vi "PXI_Host_I32_Read_NewMethod_Benchmark.vi"() -> ()   [LabVIEW 2018]
uses:
  <vilib>/Platform/TimedLoop/XDataNode/timing_clust.ctl
  <vilib>/Platform/TimedLoop/XDataNode/nitl_modes.ctl
  <vilib>/Platform/TimedLoop/XDataNode/wakeup.ctl
  cRIO RT/FPGA Bitfile Register Operations/Scalar IO Operations/Utilities/Find Register Offset.vi
  cRIO RT/FPGA Bitfile Register Operations/Scalar IO Operations/SubVIs/Check Register Data Store.vi
  cRIO RT/FPGA Bitfile Register Operations/Scalar IO Operations/Error Handling/Error 6001.vi
  cRIO RT/FPGA Bitfile Register Operations/Scalar IO Operations/Error Handling/Error 6000.vi
  cRIO RT/FPGA Bitfile Register Operations/Scalar IO Operations/Error Handling/Error 6002.vi
  cRIO RT/FPGA Bitfile Register Operations/Scalar IO Operations/Error Handling/Error 6003.vi
  <vilib>/FPGAPlugInAG/Dynamic/niLvFpga_Close_Dynamic.vi
  <vilib>/platform/TimedLoop/XDataNode/XDataNode.xnode
  <vilib>/rvi/interface/nirviCloseFPGA/nirviCloseFPGA.xnode
  cRIO RT/FPGA Bitfile Register Operations/Scalar IO Operations/Read Methods/Read Data Register/Instances/Read I32.vi
  cRIO RT/FPGA Bitfile Register Operations/Scalar IO Operations/FPGA Register IO.lvlib
  <vilib>/Platform/TimedLoop/XDataNode/XDNodeRunTimeDep.lvlib
panel:
  out "Waveform Graph":dbl[](graph)
  out "Standard Dev":dbl
  out "Arithmetic Mean":dbl
  out "Maximum":dbl
  out "Value out":i32
  out "error out":errorcluster
  # "Recorded time"
  # "3.37551E-5"
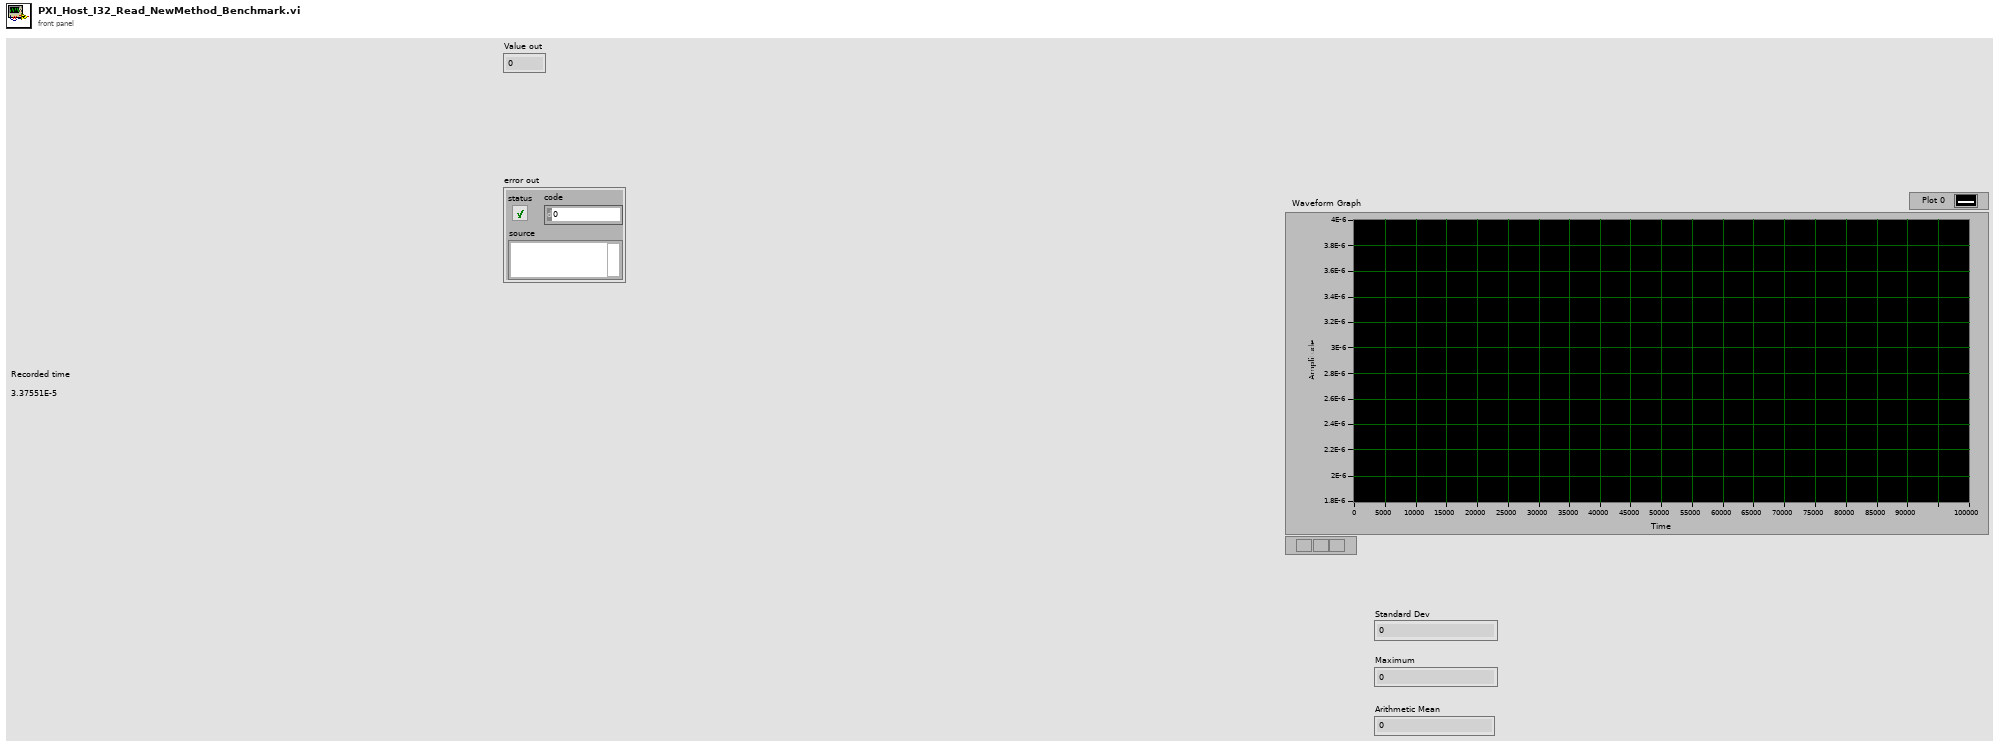
[diagram p1: front panel]
types:
  T1 = typedef "XDNodeRunTimeDep.lvlib/timing_clust.ctl" = cluster{"Expected End [f-1]":u64, "Actual End [f-1]":u64, "Finished Late? [f-1]":bool, "Expected End [i-1]":u64, "Actual End [i-1]":u64, "Finished Late? [i-1]":bool, "Expected Start [i]":u64, "Actual Start [i]":u64, "Expected Start [f]":u64, "Actual Start [f]":u64, "Source Name":string, "Structure Name":string, "Period":i64, "Deadline":i64, "Offset":i64, "Start":i64, "Priority":i32, "Timeout":i32, "Mode":T2, "Wakeup Reason":T3, "Error":errorcluster, "Source Type":string, "Secondary Source Type":string, "Global End Time":u64, "Global Start Time":u64, "Frame Duration":u64, "Iteration Duration":u64, "Assigned CPU":i32, "I/O Scan Engine Mode":u32}
  T2 = typedef "XDNodeRunTimeDep.lvlib/nitl_modes.ctl" = enum32{"No Change", "Process missed periods, maintain original phase", "Discard missed periods, maintain original phase", "Process missed periods, ignore original phase", "Discard missed periods, ignore original phase"}
  T3 = typedef "XDNodeRunTimeDep.lvlib/wakeup.ctl" = enum32{"Normal", "Aborted", "Asynchronous wakeup", "Timing source error", "Timed loop error", "Timeout"}
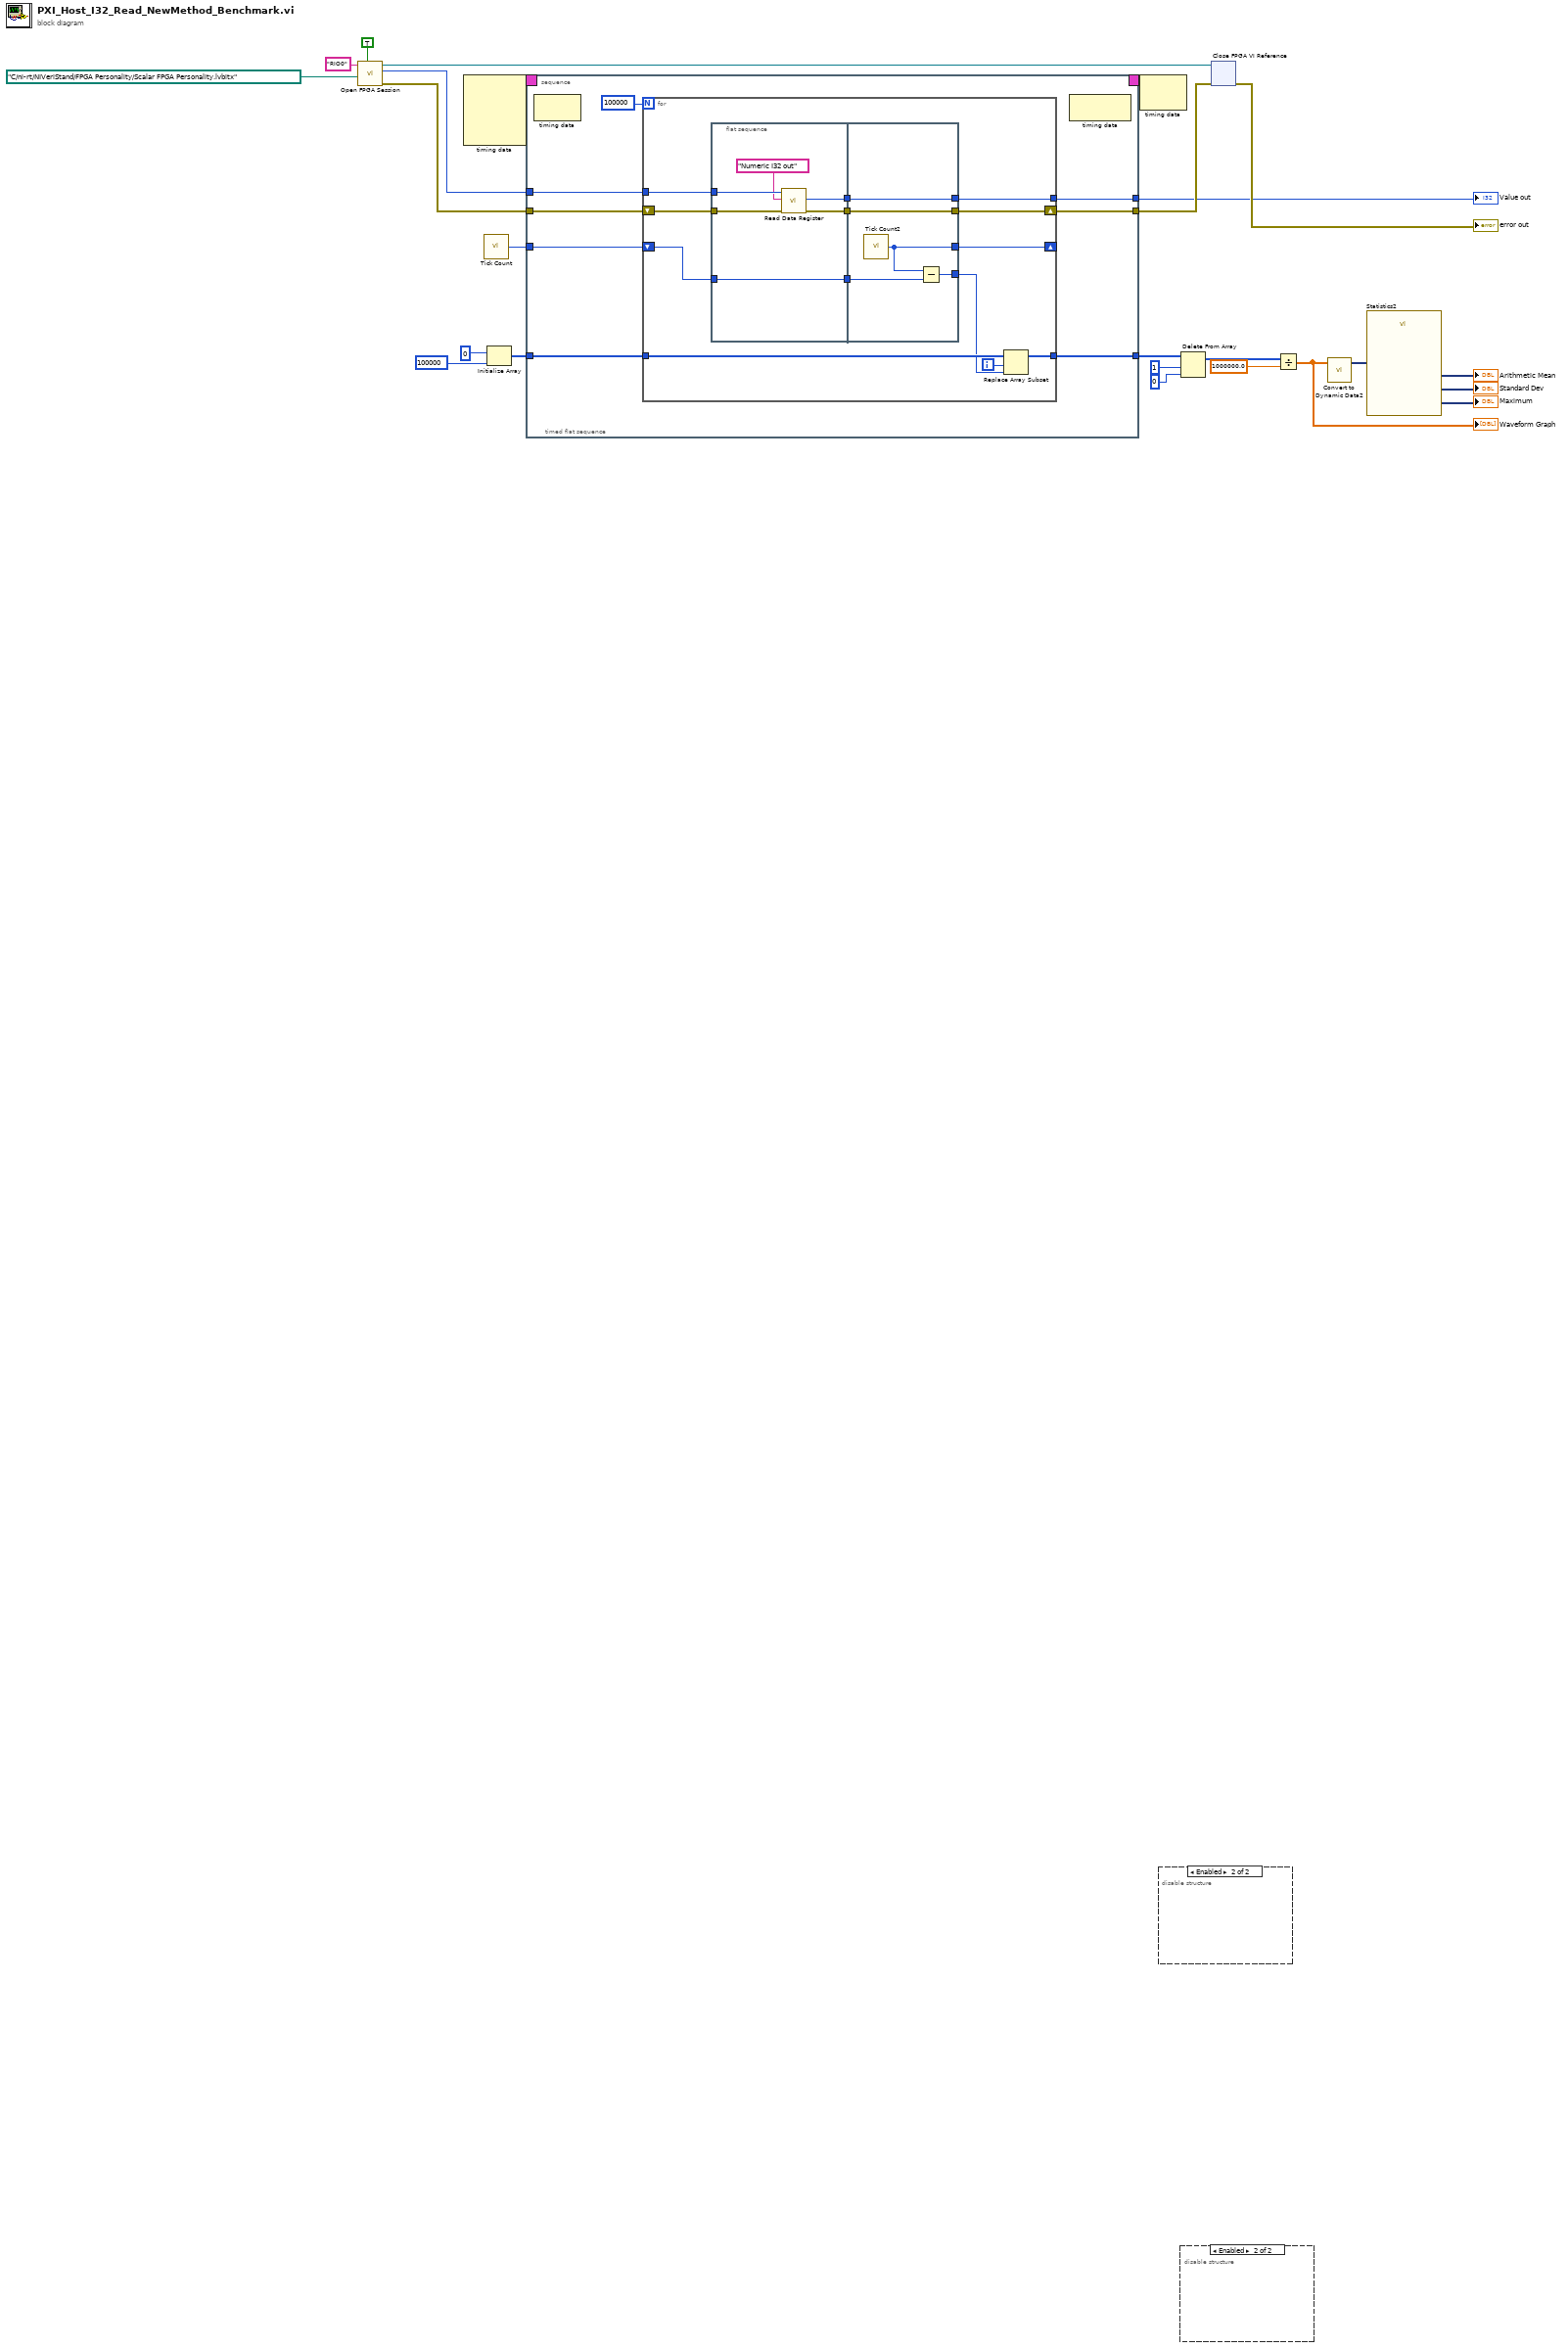
[diagram p0: block diagram]
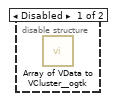
[diagram p2: hidden frame]
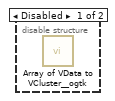
[diagram p3: hidden frame]
diagram:
  n1 = call "Open FPGA Session.vi"("run when loaded (T)"=TRUE, "bitfile path"=path "C:/ni-rt/NIVeriStand/FPGA Personality/Scalar FPGA Personality.lvbitx", "device address"="RIO0") -> ("error out"=w21:errorcluster, "session out"=w25:u32, "bitfile reference out"=w20:refnum<k20>)  [unwired: 6 in]
  n2 = node-c288() -> (w15:T1)  [unwired: 4 in]
  n3 = call "Tick Count"() -> ("Tick Count(uSec)"=w16:u32)
  n4 = Initialize Array(u32 0 ("Tick Count(uSec)"), 100000) -> (w11:u32[])
  n5 = timed-sequence {
    timing: w15 -> [_]
    timing-out: [_] -> w14
    tunnel: w25 -> [w32]
    tunnel: w21 -> [w31]
    tunnel: [w30] -> w19
    tunnel: [w29] -> w17
    tunnel: w16 -> [w28]
    tunnel: w11 -> [w27]
    tunnel: [w26] -> w1
    n6 = timed-flat-sequence {
      tunnel: w32 -> [w40]
      tunnel: w31 -> [w39]
      tunnel: [w38] -> w30
      tunnel: [w37] -> w29
      tunnel: w28 -> [w36]
      tunnel: w27 -> [w34]
      tunnel: [w33] -> w26
      n7 = node-c288() -> ()  [unwired: 1 in, 1 out]
      n8 = for {
        N: 100000 -> [_]
        tunnel: w40 -> [w52]
        tunnel: [w49] -> w37
        shift-right: [w50] -> w38
        shift-left: w39 -> [w51]
        shift-right: [w47] -> _
        shift-left: w36 -> [w48]
        tunnel: w34 -> [w46]
        tunnel: [w43] -> w33
        i -> [w45]
        n9 = flat-sequence {
          tunnel: [w59] -> w55
          tunnel: [w58] -> w54
          tunnel: w52 -> [w61]
          tunnel: w51 -> [w60]
          tunnel: w48 -> [w57]
          tunnel: [w57] -> w53
          tunnel: [w66] -> w44
          tunnel: w55 -> [w65]
          tunnel: [w65] -> w50
          tunnel: w54 -> [w64]
          tunnel: [w64] -> w49
          tunnel: w53 -> [w63]
          tunnel: [w62] -> w47
          frame #0 {
            n10 = call-poly "Read Data Register.vi"("error in"=w60, "register name"="Numeric I32 out", "session in"=w61) -> ("error out"=w59:errorcluster, "value out"=w58:i32)  [unwired: 6 in, 1 out]
          }
          frame #1 {
            n11 = call "Tick Count2"() -> ("Tick Count(uSec)"=w62:u32)
            n12 = Subtract(x=w62, y=w63) -> (x-y=w66:u32)
          }
        }
        n13 = Replace Array Subset(array=w46, new element=w44, index=w45) -> (w43:u32[])
      }
      n14 = node-c288() -> ()  [unwired: 1 in, 1 out]
    }
  }
  "Value out" <- w17
  n15 = node-c288(w14) -> ()  [unwired: 1 out]
  n16 = disable-structure shown="Enabled" {
    frame Disabled {
      n17 = call <userlib>:"Array of VData to VCluster__ogtk.vi"() -> ()  [unwired: 10 in, 2 out]
    }
    frame Enabled {
    }
  }
  n18 = disable-structure shown="Enabled" {
    frame Disabled {
      n19 = call <userlib>:"Array of VData to VCluster__ogtk.vi"() -> ()  [unwired: 10 in, 2 out]
    }
    frame Enabled {
    }
  }
  n20 = Delete From Array(array=w1, length=1, index=0) -> (array with subset deleted=w2:u32[])  [unwired: 1 out]
  n21 = xnode "Close FPGA VI Reference"("FPGA VI Reference In"=w20, "error in"=w19) -> ("error out"=→"error out":errorcluster)
  n22 = Divide(x=w2, y=1000000.0) -> (x/y=w3:dbl[])
  "Waveform Graph" <- w3
  n23 = call "Convert to Dynamic Data2"("Array"=w3) -> ("Dynamic Data Type"=w10:dynamicdata)  [unwired: 3 in]
  n24 = call "Statistics2"("Signals"=w10) -> ("Standard Dev"=→"Standard Dev":dynamicdata, "Arithmetic Mean"=→"Arithmetic Mean":dynamicdata, "Maximum"=→"Maximum":dynamicdata)  [unwired: 23 in, 1 out]
